vi "ImageGetDynamicRange.vi"(8 "error in (no error)":errorcluster, 11 "Image in":refnum<class "Image.lvclass">) -> (0 "error out":errorcluster, 3 "Image out":refnum<class "Image.lvclass">)   [LabVIEW 2012, in "Image.lvclass"]
uses:
  classes/Image.lvclass
panel:
  in  "High Range":dbl[](array[numeric])=[0.0, 0.0, 16000.0]
  in  "Low Range":dbl[](array[numeric])=[0.0, 0.0, 16000.0]
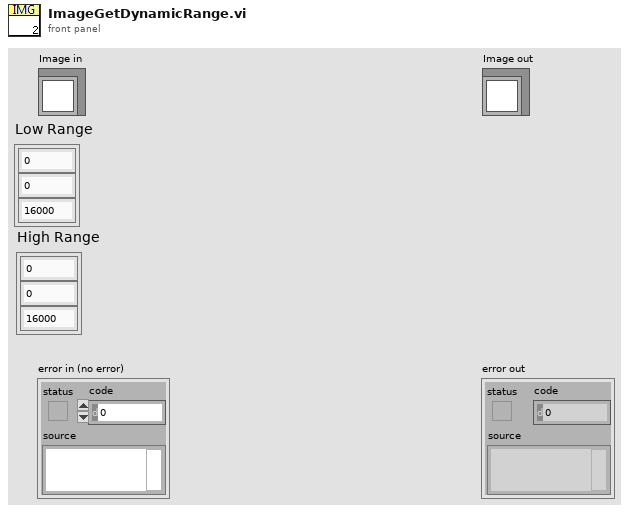
[diagram p1: front panel]
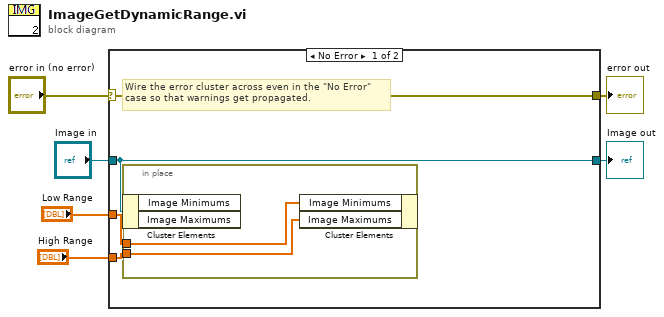
[diagram p0: block diagram]
diagram:
  n1 = case shown="No Error" "error in (no error)" {
    selector: "error in (no error)" -> [w10 w14]
    tunnel: [w10 w14] -> w5
    tunnel: [w9 w13] -> w3
    tunnel: "Image in" -> [w9 w13]
    tunnel: "Low Range" -> [w8 _]
    tunnel: "High Range" -> [w7 _]
    frame No Error {
      # "Wire the error cluster across even in the \"No Error\"\ncase so that warnings get propagated."
      n2 = in-place {
        in-place-border: w8 -> [w12]
        in-place-border: w7 -> [w11]
        n3 = in-place-cluster #1(w9) -> ()  [unwired: 2 out]
        n4 = in-place-cluster #1("Image Minimums"=w12, "Image Maximums"=w11) -> ()  [unwired: 1 out]
      }
    }
    frame Error {
    }
  }
  "error out" <- w5
  "Image out" <- w3
